vi "Drivetrain Loop.vi"() -> ()   [LabVIEW 2017]
uses:
  Common Code/Drivetrain Encoder Values.ctl
  Common Code/Drivetrain Status Cluster.ctl
  Common Code/Drivetrain Mode.ctl
  Common Code/DT Encoder Values.ctl
  Robot Global Data.vi
  <vilib>/Rock Robotics/WPI/Solenoid/Deprecated/WPI_SolenoidSetBool.vi
panel:
  out "DT Encoder Values":T1
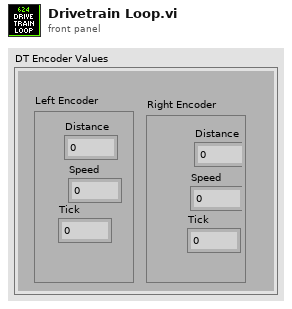
[diagram p1: front panel]
types:
  T1 = typedef "Drivetrain Encoder Values.ctl" = cluster{"Left Encoder":cluster{"Distance":dbl, "Speed":dbl, "Tick":dbl}, "Right Encoder":cluster{"Distance":dbl, "Speed":dbl, "Tick":dbl}}
  T2 = typedef "Drivetrain Status Cluster.ctl" = cluster{"Throttle (Y)":dbl, "Steer (X)":dbl, "Drivetrain Mode":T3, "Brake?":bool, "Distance Drive Complete?":bool, "PID Drive Complete?":bool, "Creep Mode?":bool, "Gyro Steer Complete?":bool, "Gyro":dbl, "X Max Output":dbl, "X Min Output":dbl, "Y Max Output ":dbl, "Y Min Output":dbl, "Heading Target":dbl, "Distance Target":dbl, "2nd Gear":bool, "Drivetrain Encoder Values":T4}
  T3 = typedef "Drivetrain Mode.ctl" = enum16{"Manual", "Gyro Steer", "PID Drive", "Distance Drive", "Autonomous"}
  T4 = typedef "DT Encoder Values.ctl" = cluster{"Left Encoder":cluster{"Distance":dbl, "Speed":dbl, "Tick":dbl}, "Right Encoder":cluster{"Distance":dbl, "Speed":dbl, "Tick":dbl}}
  T5 = typedef "Dashboard Control Data.ctl" = cluster{"Drivetrain Settings Cluster":T6, "Intake Presets":T8, "Elevator Settings Cluster":T9, "Zero All?":bool}
  T6 = typedef "Drivetrain Settings Cluster.ctl" = cluster{"Gyro Steer PID Gains":T7, "Distance Drive PID Gains":T7, "Drive Tolerance":dbl, "Gyro Tolerance":dbl, "Gyro Output":dbl, "Distance Output":dbl, "Y Power Multiplier":dbl, "Turn Power Multiplier":dbl, "Creep Rate":dbl, "Constant Power":bool, "DT Mode Modifier":enum16{"None, Default", "Cube", "Square"}, "Left Encoder Tick Constant":dbl, "Right Encoder Tick Constant":dbl, "Shift Speed":dbl}
  T7 = typedef "PID Gains Cluster.ctl" = cluster{"Integral Time":dbl, "Proportional Gain":dbl, "Derivative Time":dbl}
  T8 = typedef "Intake Presets.ctl" = cluster{"Idle Angle":dbl, "Mid Angle":dbl, "Low Angle":dbl, "Outtake Power":dbl, "Intake Power":dbl, "Unstuck":dbl, "Angle Tolerance":dbl, "Max Angle":dbl, "Max Current":dbl, "Current Trip Time":dbl, "Reset Encoder?":bool, "Encoder Scale":dbl, "PID gains":cluster{"proportional gain (Kc)":dbl, "integral time (Ti, min)":dbl, "derivative time (Td, min)":dbl}, "output range":cluster{"output high":dbl, "output low":dbl}}
  T9 = typedef "Elevator Settings Cluster.ctl" = cluster{"Ground Height":dbl, "Switch Height":dbl, "Scale High Height ":dbl, "Scale Low Height":dbl, "Elevator PID Gains":T10, "Elevator Tolerance":dbl, "Reset Encoders":bool, "Encoder Scale":dbl, "Max Height":dbl, "Mid Height":dbl, "output range":cluster{"output high":dbl, "output low":dbl}}
  T10 = typedef "PID Gains.ctl" = cluster{"proportional gain (Kc)":dbl, "integral time (Ti, min)":dbl, "derivative time (Td, min)":dbl}
  T11 = typedef "Drivetrain Command Cluster.ctl" = cluster{"Y Power":dbl, "Turn Power":dbl, "Drivetrain Mode":T3, "Gear 2":bool, "Y Min Output":dbl, "Y Max Output":dbl, "X Min Output":dbl, "X Max Output":dbl, "Heading Target":dbl, "Distance Target":dbl, "Brake?":bool}
  T12 = cluster{"Target Heading":dbl, "Target Distance":dbl}
  T13 = cluster{"Y Max Output":dbl, "Y Min Output":dbl, "X Min Output":dbl, "X Max Output":dbl}
  T14 = cluster{"Distance Tolerance":dbl, "Gyro Tolerance":dbl}
  T15 = typedef "WPI_MotorControlDeviceRef.ctl" = cluster{"DeviceStatus":errorcluster, "Type":T16, "PWM":cluster{"PWM Channel":T17, "DeadBand":T18}, "CAN":cluster{"Device Number":u8, "SetOutput VI Ref":variant, "GetOutput VI Ref":variant, "Enable VI Ref":variant, "Disable VI Ref":variant, "Data":variant}, "Invert":bool, "DIO PWM":cluster{"PWM \"Enable\" Channel":T17, "DIOChannel":T19, "PWM Rate":dbl}}
  T16 = typedef "WPI_MotorControlType.ctl" = enum16{"PWM", "CAN", "DIO PWM"}
  T17 = typedef "FPGA_DIOPWMChannel.ctl" = enum8{"PWM 0", "PWM 1", "PWM 2", "PWM 3", "PWM 4", "PWM 5", "PWM 6", "PWM 7", "PWM 8", "PWM 9", "PWM MXP 0", "PWM MXP 1", "PWM MXP 2", "PWM MXP 3", "PWM MXP 4", "PWM MXP 5", "PWM MXP 6", "PWM MXP 7", "PWM MXP 8", "PWM MXP 9", "Invalid"}
  T18 = typedef "WPI_PWMDeadband.ctl" = cluster{"Name":string, "maxPositivePwm":i32, "minPositivePwm":i32, "centerPwm":i32, "maxNegativePwm":i32, "minNegativePwm":i32, "angularRange":u16}
  T19 = typedef "FPGA_DIOChannel.ctl" = enum8{"DIO 0", "DIO 1", "DIO 2", "DIO 3", "DIO 4", "DIO 5", "DIO 6", "DIO 7", "DIO 8", "DIO 9", "DIO MXP 0", "DIO MXP 1", "DIO MXP 2", "DIO MXP 3", "DIO MXP 4", "DIO MXP 5", "DIO MXP 6", "DIO MXP 7", "DIO MXP 8", "DIO MXP 9", "DIO MXP 10", "DIO MXP 11", "DIO MXP 12", "DIO MXP 13", "DIO MXP 14", "DIO MXP 15", "SPI Port CS1", "SPI Port CS2", "SPI Port CS3", "SPI Port MISO", "SPI Port MOSI", "Invalid"}
  T20 = typedef "WPI_SolenoidDevRef.ctl" = cluster{"DevStatus":errorcluster, "Pneumatics Control Module":u8, "Forward Solenoid Channel":T21, "Reverse Solenoid Channel":T21}
  T21 = typedef "WPI_SolenoidChannel.ctl" = enum8{"Solenoid 0", "Solenoid 1", "Solenoid 2", "Solenoid 3", "Solenoid 4", "Solenoid 5", "Solenoid 6", "Solenoid 7", "Invalid"}
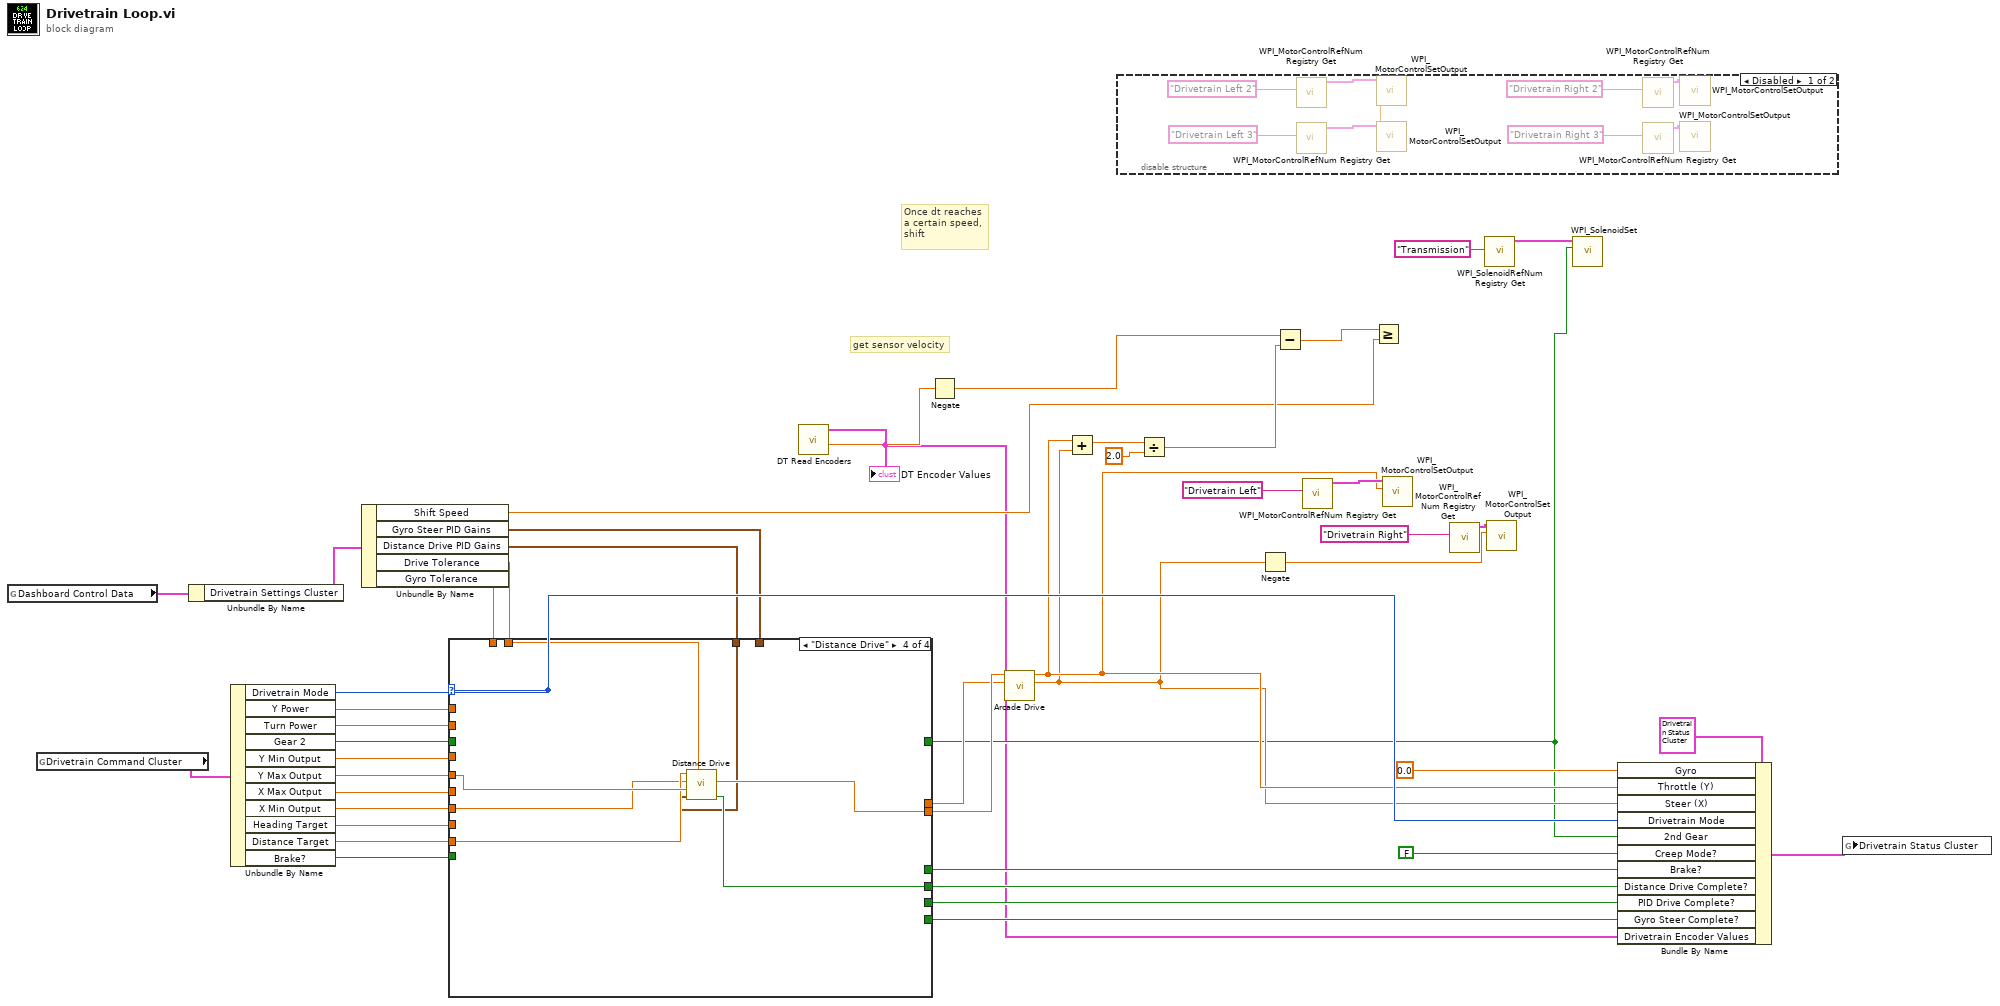
[diagram p0: block diagram]
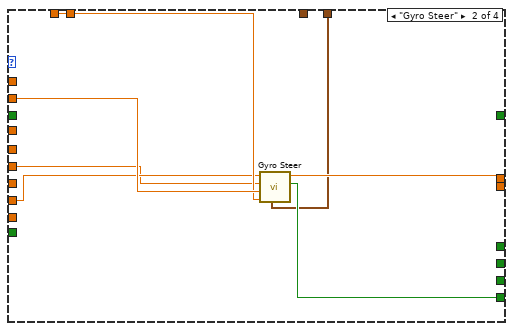
[diagram p4: hidden frame]
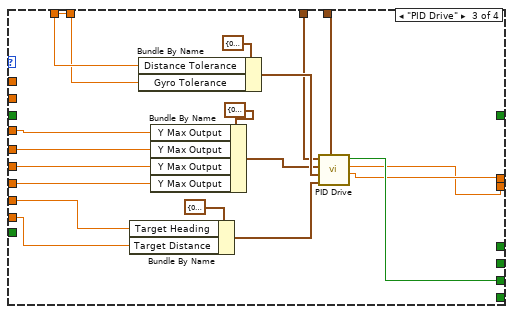
[diagram p5: hidden frame]
diagram:
  # "get sensor velocity"
  # "Once dt reaches\na certain speed,\nshift"
  n1 = global read "Robot Global Data.vi" "Dashboard Control Data"() -> (w15:T5)
  n2 = global read "Robot Global Data.vi" "Drivetrain Command Cluster"() -> (w23:T11)
  n3 = Unbundle By Name(w15) -> ("Drivetrain Settings Cluster"=w16:T6)
  n4 = Unbundle By Name(w23) -> ("Drivetrain Mode"=w34:T3, "Y Power"=w33:dbl, "Turn Power"=w32:dbl, "Gear 2"=w31:bool, "Y Min Output"=w30:dbl, "Y Max Output"=w29:dbl, "X Max Output"=w28:dbl, "X Min Output"=w27:dbl, "Heading Target"=w26:dbl, "Distance Target"=w25:dbl, "Brake?"=w24:bool)
  n5 = Unbundle By Name(w16) -> ("Shift Speed"=w5:dbl, "Gyro Steer PID Gains"=w18:T7, "Distance Drive PID Gains"=w17:T7, "Drive Tolerance"=w14:dbl, "Gyro Tolerance"=w13:dbl)
  n6 = case shown="\"Distance Drive\"" w34 {
    tunnel: w33 -> [w49 _ _ _]
    tunnel: w32 -> [w50 w57 _ _]
    tunnel: [w49 _ w58 w79] -> w40
    tunnel: [w50 w55 w61 _] -> w39
    tunnel: w31 -> [w47 _ _ _]
    tunnel: [_ _ w62 _] -> w37
    tunnel: [_ _ _ w80] -> w36
    tunnel: [w48 _ _ _] -> w35
    tunnel: w30 -> [_ _ w76 _]
    tunnel: w29 -> [_ _ w75 w83]
    tunnel: w25 -> [_ _ w74 w82]
    tunnel: w24 -> [w48 _ _ _]
    tunnel: w27 -> [_ _ w73 w81]
    tunnel: w28 -> [_ w51 w72 _]
    tunnel: w26 -> [_ w52 w71 _]
    tunnel: [_ w56 _ _] -> w22
    tunnel: w14 -> [_ _ w70 w78]
    tunnel: w17 -> [_ _ w60 w77]
    tunnel: w13 -> [_ w54 w68 _]
    tunnel: w18 -> [_ w53 w59 _]
    tunnel: [w47 _ _ _] -> w2
    frame "Manual", Default {
    }
    frame "Gyro Steer" {
      n7 = call "Gyro Steer.vi"("Steer PID Gains"=w53, "Gyro Tolerance"=w54, "X Min Output"=w57, "X Max Output"=w51, "Target Heading"=w52) -> ("Finished"=w56:bool, "X Out"=w55:dbl)  [unwired: 5 in]
    }
    frame "PID Drive" {
      n8 = Bundle By Name(cluster=T12 {"Target Heading"=0.0, "Target Distance"=0.0} ("input cluster"), "Target Heading"=w71, "Target Distance"=w74) -> (w64:T12)
      n9 = Bundle By Name(cluster=T14 {"Distance Tolerance"=0.0, "Gyro Tolerance"=0.0} ("Tolerances"), "Distance Tolerance"=w70, "Gyro Tolerance"=w68) -> (w69:T14)
      n10 = Bundle By Name(cluster=T13 {"Y Max Output"=0.0, "Y Min Output"=0.0, "X Min Output"=0.0, "X Max Output"=0.0} ("input cluster"), "Y Max Output"=w76, "Y Max Output"=w75, "Y Max Output"=w72, "Y Max Output"=w73) -> (w66:T13)
      n11 = call "PID Drive.vi"("Steer PID Gains"=w59, "Targets"=w64, "Tolerances"=w69, "Motor Values"=w66, "Drive PID Gains"=w60) -> ("Y Out"=w61:dbl, "X Out"=w58:dbl, "Finished?"=w62:bool)  [unwired: 4 in]
    }
    frame "Distance Drive" {
      n12 = call "Distance Drive.vi"("Distance Tolerance"=w78, "Drive PID Gains"=w77, "Y Max Output"=w83, "Y Min Output"=w81, "Distance Target"=w82) -> ("Finished"=w80:bool, "Y Output"=w79:dbl)  [unwired: 5 in]
    }
  }
  n13 = call "DT Read Encoders.vi"() -> ("Rate"=w12:dbl, "DT Encoder Values"=w1:T1)  [unwired: 10 in]
  "DT Encoder Values" <- w1
  n14 = Negate(x=w12) -> (-x=w7:dbl)
  n15 = call "Arcade Drive.vi"("Turn Power"=w39, "Y Power"=w40) -> ("Right Motor Output"=w4:dbl, "Left Motor Output"=w11:dbl)  [unwired: 8 in]
  n16 = Add(x=w11, y=w4) -> (x+y=w10:dbl)
  n17 = disable-structure shown="Disabled" {
    frame Disabled {
      n18 = call <vilib>:"WPI_MotorControlRefNum Registry Get.vi"("refnum name"="Drivetrain Left 2") -> ("MotorControlDevRef"=w94:T15)  [unwired: 9 in, 1 out]
      n19 = call <vilib>:"WPI_MotorControlRefNum Registry Get.vi"("refnum name"="Drivetrain Left 3") -> ("MotorControlDevRef"=w93:T15)  [unwired: 9 in, 1 out]
      n20 = call <vilib>:"WPI_MotorControlSetOutput.vi"("MotorControlDevRef"=w93) -> ("Output"=w85:dbl)  [unwired: 7 in, 3 out]
      n21 = call <vilib>:"WPI_MotorControlSetOutput.vi"("Output"=w85, "MotorControlDevRef"=w94) -> ()  [unwired: 7 in, 3 out]
      n22 = call <vilib>:"WPI_MotorControlRefNum Registry Get.vi"("refnum name"="Drivetrain Right 2") -> ("MotorControlDevRef"=w90:T15)  [unwired: 9 in, 1 out]
      n23 = call <vilib>:"WPI_MotorControlRefNum Registry Get.vi"("refnum name"="Drivetrain Right 3") -> ("MotorControlDevRef"=w89:T15)  [unwired: 9 in, 1 out]
      n24 = call <vilib>:"WPI_MotorControlSetOutput.vi"("MotorControlDevRef"=w90) -> ("Output"=w84:dbl)  [unwired: 7 in, 3 out]
      n25 = call <vilib>:"WPI_MotorControlSetOutput.vi"("MotorControlDevRef"=w89) -> ("Output"=w86:dbl)  [unwired: 7 in, 3 out]
    }
    frame Enabled {
    }
  }
  n26 = Divide(x=w10, y=2.0) -> (x/y=w8:dbl)
  n27 = Negate(x=w4) -> (-x=w3:dbl)
  n28 = Subtract(x=w7, y=w8) -> (x-y=w6:dbl)
  n29 = call <vilib>:"WPI_MotorControlRefNum Registry Get.vi"("refnum name"="Drivetrain Left") -> ("MotorControlDevRef"=w46:T15)  [unwired: 9 in, 1 out]
  n30 = Greater Or Equal?(x=w6, y=w5) -> ()  [unwired: 1 out]
  n31 = call <vilib>:"WPI_MotorControlSetOutput.vi"("Output"=w11, "MotorControlDevRef"=w46) -> ()  [unwired: 7 in, 3 out]
  n32 = call <vilib>:"WPI_MotorControlRefNum Registry Get.vi"("refnum name"="Drivetrain Right") -> ("MotorControlDevRef"=w42:T15)  [unwired: 9 in, 1 out]
  n33 = call <vilib>:"WPI_SolenoidRefNum Registry Get.vi"("refnum name"="Transmission") -> ("SolenoidDevRef"=w44:T20)  [unwired: 9 in, 1 out]
  n34 = call <vilib>:"WPI_MotorControlSetOutput.vi"("Output"=w3, "MotorControlDevRef"=w42) -> ()  [unwired: 7 in, 3 out]
  n35 = call-poly <vilib>:"WPI_SolenoidSet.vi"("Value"=w2, "SolenoidDevRef"=w44) -> ()  [unwired: 8 in, 2 out]
  n36 = Bundle By Name(cluster=T2 {"Throttle (Y)"=0.0, "Steer (X)"=0.0, "Drivetrain Mode"=enum."Manual", "Brake?"=FALSE, "Distance Drive Complete?"=FALSE, "PID Drive Complete?"=FALSE, "Creep Mode?"=FALSE, "Gyro Steer Complete?"=FALSE, "Gyro"=0.0, "X Max Output"=0.0, "X Min Output"=0.0, "Y Max Output "=0.0, "Y Min Output"=0.0, "Heading Target"=0.0, "Distance Target"=0.0, "2nd Gear"=FALSE, "Drivetrain Encoder Values"={"Left Encoder"={"Distance"=0.0, "Speed"=0.0, "Tick"=0.0}, "Right Encoder"={"Distance"=0.0, "Speed"=0.0, "Tick"=0.0}}} ("Drivetrain Status Cluster"), "Gyro"=0.0, "Throttle (Y)"=w11, "Steer (X)"=w4, "Drivetrain Mode"=w34, "2nd Gear"=w2, "Creep Mode?"=FALSE, "Brake?"=w35, "Distance Drive Complete?"=w36, "PID Drive Complete?"=w37, "Gyro Steer Complete?"=w22, "Drivetrain Encoder Values"=w1) -> (w38:T2)
  n37 = global write "Robot Global Data.vi" "Drivetrain Status Cluster"(w38) -> ()
